vi "HAPS_PhaseSweep_Preamp(Hz).vi"() -> ()   [LabVIEW 2023, in "HAPS.lvlib"]
uses:
  HAPS.lvlib
  MCU_Function.ctl
  set_ele.ctl
  HAPS_SerialPort.ctl
  HAPS_MCU_ELE_Func.ctl
  R_S/R_S.lvlib
panel:
  in  "IC_On/OFF":bool[][](array[boolean])=[[TRUE, TRUE, TRUE, TRUE, TRUE, TRUE, FALSE, FALSE, FALSE, FALSE, FALSE, FALSE, TRUE], [FALSE, FALSE, FALSE, FALSE, FALSE, FALSE, FALSE, FALSE, FALSE, FALSE, FALSE, FALSE, FALSE], [FALSE, FALSE, FALSE, FALSE, FALSE, FALSE, TRUE, TRUE, TRUE, TRUE, TRUE, FALSE, TRUE]]
  in  "comn_gain":i32=17
  in  "ele_gain":i32=35
  in  "File_note":string
  in  "Init?":bool=TRUE
  out "Duration":dbl
  out "In-Phase : Phase(degree)":dbl[](graph)
  out "In-Phase : Gain(dB)":dbl[](graph)
  out "channel":i32
  out "chain_id":i32
  out "group":i32
  out "array_id":i32
  in  "Tx/Rx":enum16{"Rx", "Tx"}(ring)=enum."Tx"
  in  "array_id (MCU index)":i32
  in  "MCU_UART_addr":refnum<visa-resource-name>="COM8"
  in  "Target(degree)":dbl format="%#_13g"
  in  "SweepPoints":i32=11
  in  "sParameter":i32=21
  in  "Stop_Freq(GHz)":i64=39000000250
  in  "Start_Freq(GHz)":i64=38999999750
  in  "VISA resource name":refnum<visa-resource-name>="TCPIP0::192.168.119.45::inst0::INSTR"
  in  "HAPS_Equipment":enum16{"Keysight", "R&S"}(ring)=enum."R&S"
  # "HAPS_24x24_Phase_Sweep_Preamp(Hz)"
  # "VNA"
  # "DUT"
  # "Tx:35\nRx:22"
  # "4718.54"
  # "TCPIP0::192.168.1.31::hislip0::INSTR"
  # "Group_0"
  # "Group_1"
  # "Group_2"
  # "0"
  # "5"
  # "6"
  # "11"
  # "Test Status"
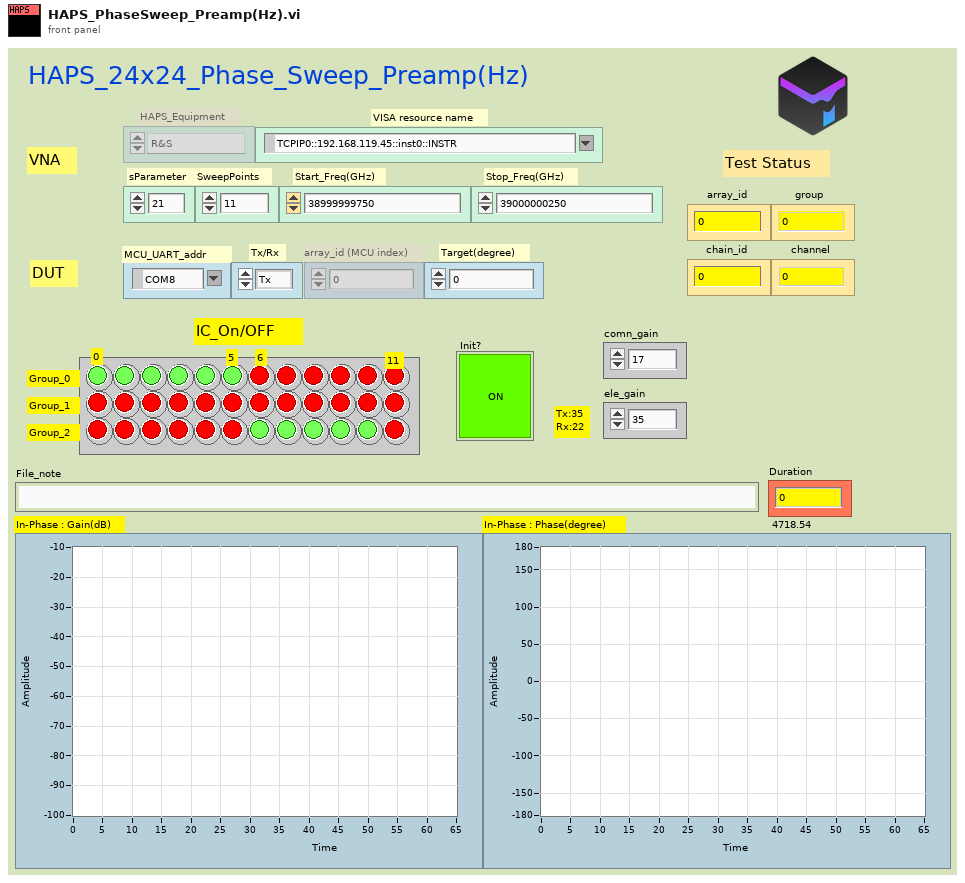
[diagram p1: front panel]
types:
  T1 = typedef "HAPS.lvlib/HAPS_SerialPort.ctl" = enum16{"Init", "Close", "CMD", "Flush"}
  T2 = typedef "HAPS.lvlib/HAPS_MCU_ELE_Func.ctl" = enum16{"array_init", "set_com_gain", "set_ch_gain_phase", "set_pd_range", "get_preamp_temp", "get_bfic_temp", "get_tx_pd", "ch_on", "ch_on_2", "ch_ctrl_all", "array_ctrl_src"}
  T3 = typedef "HAPS.lvlib/MCU_Function.ctl" = cluster{"Tx/Rx":enum16{"Rx", "Tx"}, "Enable?":enum16{"OFF", "On"}, "Source":enum16{"MCU", "ACU"}}
  T4 = typedef "HAPS.lvlib/set_ele.ctl" = cluster{"ch":i32, "chain_id":i32, "group":i32, "array_id":i32, "ele_phase":i32, "ele_gain":i32, "com_gain":i32, "pd_range":i32}
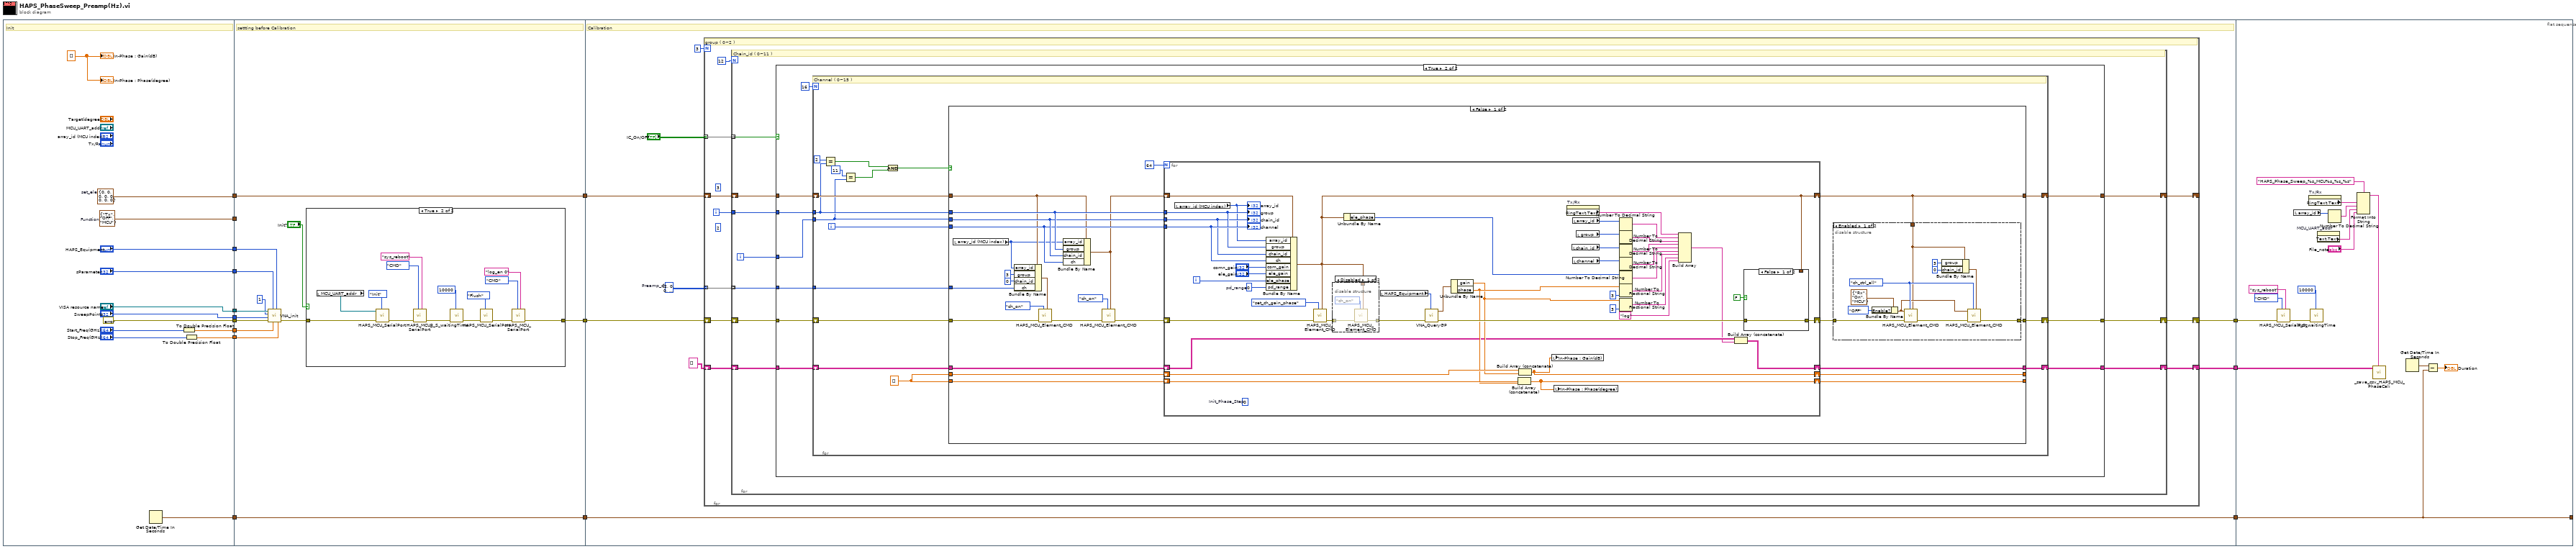
[diagram p0: block diagram]
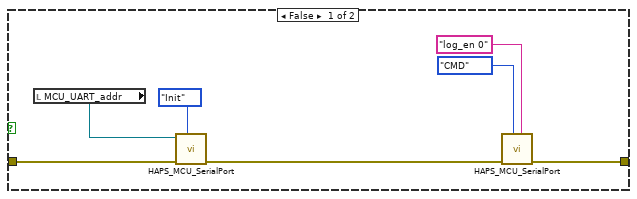
[diagram p2: hidden frame]
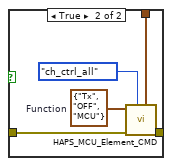
[diagram p6: hidden frame]
diagram:
  n1 = flat-sequence {
    tunnel: [w22] -> w16
    tunnel: [w29] -> w15
    tunnel: [errorcluster {"status"=FALSE, "code"=0, "source"=""} ("error in")] -> w13
    tunnel: ["sParameter"] -> w11
    tunnel: ["VISA resource name"] -> w10
    tunnel: [w18] -> w9
    tunnel: [w17] -> w8
    tunnel: ["SweepPoints"] -> w7
    tunnel: ["HAPS_Equipment"] -> w6
    tunnel: [w19] -> w4
    tunnel: w16 -> [w42]
    tunnel: w15 -> [_]
    tunnel: [w42] -> w14
    tunnel: w13 -> [w41]
    tunnel: [w33] -> w12
    tunnel: w11 -> [w40]
    tunnel: w10 -> [w39]
    tunnel: w9 -> [w38]
    tunnel: w8 -> [w37]
    tunnel: w7 -> [w36]
    tunnel: w6 -> [w32]
    tunnel: [w31] -> w5
    tunnel: w4 -> [w31]
    tunnel: w14 -> [w71]
    tunnel: w12 -> [w72]
    tunnel: w5 -> [w68]
    tunnel: [w68] -> w3
    tunnel: [w67] -> w2
    tunnel: [w65] -> w1
    tunnel: [w226] -> _
    tunnel: w3 -> [w226]
    tunnel: w2 -> [w228]
    tunnel: w1 -> [w221]
    frame #0 {
      w20 = dbl[] []
      w22 = T4 {"ch"=0, "chain_id"=0, "group"=0, "array_id"=0, "ele_phase"=0, "ele_gain"=0, "com_gain"=0, "pd_range"=0}  # set_ele
      w29 = T3 {"Tx/Rx"=enum."Tx", "Enable?"=enum."OFF", "Source"=enum."MCU"}  # Function
      # "Init"
      n2 = Get Date/Time In Seconds() -> (seconds since 1Jan1904=w19:timestamp)
      n3 = To Double Precision Float(number="Start_Freq(GHz)") -> (double precision float=w18:dbl)
      n4 = To Double Precision Float(number="Stop_Freq(GHz)") -> (double precision float=w17:dbl)
      "In-Phase : Gain(dB)" <- w20
      "In-Phase : Phase(degree)" <- w20
    }
    frame #1 {
      # "settting before Calibration"
      n5 = call "VNA_init.vi"("Stop_Freq(GHz)"=w37, "HAPS_MCU_CMD"=w32, "Start_Freq(GHz)"=w38, "sParameter"=w40, "error in"=w41, "SweepPoints"=w36, "Mark no."=1, "VISA resource name"=w39) -> ("error out"=w34:errorcluster)  [unwired: 3 in]
      n6 = case shown="True" "Init?" {
        tunnel: w34 -> [w47 w61]
        tunnel: [w44 w58] -> w33
        frame False {
          n7 = local read "MCU_UART_addr"() -> (w45:refnum<visa-resource-name>)
          n8 = call "HAPS_MCU_SerialPort.vi"("HAPS_SerialPort_Func"=HAPS_SerialPort."Init", "error in"=w47, "VISA resource name"=w45) -> ("error out"=w43:errorcluster)  [unwired: 6 in, 2 out]
          n9 = call "HAPS_MCU_SerialPort.vi"("Command"="log_en 0", "HAPS_SerialPort_Func"=enum16{"Init", "Close", "CMD"}."CMD" ("HAPS_SerialPort"), "error in"=w43) -> ("error out"=w44:errorcluster)  [unwired: 6 in, 2 out]
        }
        frame True {
          n10 = local read "MCU_UART_addr"() -> (w59:refnum<visa-resource-name>)
          n11 = call "HAPS_MCU_SerialPort.vi"("HAPS_SerialPort_Func"=HAPS_SerialPort."Init", "error in"=w61, "VISA resource name"=w59) -> ("error out"=w55:errorcluster)  [unwired: 6 in, 2 out]
          n12 = call "HAPS_MCU_SerialPort.vi"("Command"="sys_reboot", "HAPS_SerialPort_Func"=enum16{"Init", "Close", "CMD"}."CMD" ("HAPS_SerialPort"), "error in"=w55) -> ("error out"=w54:errorcluster)  [unwired: 6 in, 2 out]
          n13 = call "R_S_waitingTime.vi"("Waiting Time(ms)"=u32 10000, "error in"=w54) -> ("error out"=w52:errorcluster)  [unwired: 9 in]
          n14 = call "HAPS_MCU_SerialPort.vi"("HAPS_SerialPort_Func"=HAPS_SerialPort."Flush", "error in"=w52) -> ("error out"=w50:errorcluster)  [unwired: 7 in, 2 out]
          n15 = call "HAPS_MCU_SerialPort.vi"("Command"="log_en 0", "HAPS_SerialPort_Func"=enum16{"Init", "Close", "CMD"}."CMD" ("HAPS_SerialPort"), "error in"=w50) -> ("error out"=w58:errorcluster)  [unwired: 6 in, 2 out]
        }
      }
    }
    frame #2 {
      w66 = i32[][] [[2, 0, 0, 8, 8, 10, 11, 9, 9, 1, 1, 3], [3, 1, 1, 9, 9, 11, 13, 15, 15, 7, 7, 5], [5, 7, 7, 15, 15, 13, 14, 14, 6, 6, 4, 12]]  # Preamp_ch
      # "Calibration"
      n16 = for {
        N: 3 -> [_]
        shift-right: [w82] -> _
        shift-left: w71 -> [w78]
        shift-right: [w81] -> w67
        shift-left: string[][] [] -> [w77]
        shift-right: [w80] -> w65
        shift-left: w72 -> [w79]
        tunnel: w66 -> [w74] mode=indexing
        tunnel: "IC_On/OFF" -> [w73] mode=indexing
        i -> [w75]
        (unwired) 2
        (unwired) 3
        # "group ( 0~2 )"
        n17 = for {
          N: 12 -> [_]
          shift-right: [w92] -> w82
          shift-left: w78 -> [w89]
          shift-right: [w91] -> w81
          shift-left: w77 -> [w88]
          shift-right: [w85] -> w80
          shift-left: w79 -> [w90]
          tunnel: w75 -> [w87]
          tunnel: w74 -> [w84] mode=indexing
          tunnel: w73 -> [w83] mode=indexing
          i -> [w86]
          # "Chain_id ( 0~11 )"
          n18 = case shown="True" w83 {
            tunnel: [w93 w104] -> w92
            tunnel: [w95 w103] -> w91
            tunnel: w90 -> [w94 w102]
            tunnel: w89 -> [w93 w101]
            tunnel: w88 -> [w95 w100]
            tunnel: w87 -> [_ w99]
            tunnel: w86 -> [_ w98]
            tunnel: [w94 w97] -> w85
            tunnel: w84 -> [_ w96]
            frame False {
            }
            frame True {
              n19 = for {
                N: 16 -> [_]
                shift-right: [w118] -> w104
                shift-left: w101 -> [w121]
                shift-right: [w116] -> w103
                shift-left: w100 -> [w117]
                shift-right: [w119] -> w97
                shift-left: w102 -> [w120]
                tunnel: w99 -> [w115]
                tunnel: w98 -> [w107]
                tunnel: w96 -> [w106]
                i -> [w108]
                w109 = dbl[] []
                # "Channel ( 0~15 )"
                n20 = Equal?(x=2, y=w115) -> (x = y?=w112:bool)
                n21 = Equal?(x=11, y=w107) -> (x = y?=w111:bool)
                n22 = And(x=w112, y=w111) -> (x .and. y?=w110:bool)
                n23 = case shown="False" w110 {
                  tunnel: w121 -> [w128 w215]
                  tunnel: w108 -> [w137 _]
                  tunnel: w120 -> [w129 w214]
                  tunnel: w115 -> [w139 _]
                  tunnel: w107 -> [w138 _]
                  tunnel: w109 -> [w146 w217]
                  tunnel: w109 -> [w145 w218]
                  tunnel: [w144 w217] -> _
                  tunnel: [w143 w218] -> _
                  tunnel: [w133 w214] -> w119
                  tunnel: [w132 w215] -> w118
                  tunnel: w117 -> [w141 w216]
                  tunnel: [w140 w216] -> w116
                  tunnel: w106 -> [w122 _]
                  frame False {
                    n24 = local read "array_id (MCU index)"() -> (w126:i32)
                    n25 = Bundle By Name(cluster=w128, "array_id"=w126, "group"=3, "chain_id"=0, "ch"=w122) -> (w127:T4)
                    n26 = call "HAPS_MCU_Element_CMD.vi"("set_ele"=w127, "HAPS_MCU_ELE_Func."=HAPS_MCU_ELE_Func."ch_on", "error in"=w129) -> ("error out"=w130:errorcluster)  [unwired: 7 in, 1 out]
                    n27 = Bundle By Name(cluster=w128, "array_id"=w126, "group"=w139, "chain_id"=w138, "ch"=w137) -> (w123:T4)
                    n28 = call "HAPS_MCU_Element_CMD.vi"("set_ele"=w123, "HAPS_MCU_ELE_Func."=HAPS_MCU_ELE_Func."ch_on", "error in"=w130) -> ("error out"=w135:errorcluster)  [unwired: 7 in, 1 out]
                    n29 = for {
                      N: 64 -> [_]
                      tunnel: w137 -> [w201]
                      tunnel: w139 -> [w199]
                      tunnel: w138 -> [w198]
                      shift-right: [w174] -> w144
                      shift-left: w146 -> [w176]
                      shift-right: [w173] -> w143
                      shift-left: w145 -> [w175]
                      shift-right: [w170] -> w134
                      shift-left: w135 -> [w200]
                      shift-right: [w160] -> w132
                      shift-left: w123 -> [w202]
                      shift-right: [w164] -> w140
                      shift-left: w141 -> [w166]
                      i -> [w172]
                      w196 = 0  # pd_range
                      (unwired) 0  # Init_Phase_Step
                      n30 = local read "array_id (MCU index)"() -> (w194:i32)
                      "array_id" <- w194
                      n31 = Bundle By Name(cluster=w202, "array_id"=w194, "group"=w199, "chain_id"=w198, "ch"=w201, "com_gain"="comn_gain", "ele_gain"="ele_gain", "ele_phase"=w172, "pd_range"=w196) -> (w160:T4)
                      n32 = call "HAPS_MCU_Element_CMD.vi"("set_ele"=w160, "HAPS_MCU_ELE_Func."=HAPS_MCU_ELE_Func."set_ch_gain_phase", "error in"=w200) -> ("error out"=w162:errorcluster)  [unwired: 7 in, 1 out]
                      n33 = disable-structure shown="Disabled" {
                        disable-tunnel: w162 -> [w206 w207]
                        disable-tunnel: [w205 w207] -> w161
                        disable-tunnel: w160 -> [w203 _]
                        frame Disabled {
                          n34 = call "HAPS_MCU_Element_CMD.vi"("set_ele"=w203, "HAPS_MCU_ELE_Func."=HAPS_MCU_ELE_Func."ch_on", "error in"=w206) -> ("error out"=w205:errorcluster)  [unwired: 7 in, 1 out]
                        }
                        frame Enabled {
                        }
                      }
                      n35 = Unbundle By Name(w160) -> ("ele_phase"=w169:i32)
                      n36 = local read "HAPS_Equipment"() -> (w178:enum16{"Keysight", "R&S"})
                      n37 = call "VNA_QueryGP.vi"("HAPS_Equipment"=w178, "error in"=w161) -> ("error out"=w171:errorcluster, "queryMarker"=w177:cluster{"gain":dbl, "phase":dbl})  [unwired: 8 in]
                      n38 = Unbundle By Name(w177) -> ("gain"=w167:dbl, "phase"=w168:dbl)
                      n39 = Build Array (concatenate)(w175, w168) -> (w173:dbl[])
                      n40 = Build Array (concatenate)(w176, w167) -> (w174:dbl[])
                      n41 = local write "In-Phase : Gain(dB)"(w174) -> ()
                      n42 = local write "In-Phase : Phase(degree)"(w173) -> ()
                      n43 = property on="Tx/Rx" class="Enum (strict)"() -> ("RingText.Text"=w183:string)  [unwired: 2 in, 2 out]
                      n44 = local read "chain_id"() -> (w180:i32)
                      n45 = local read "array_id"() -> (w182:i32)
                      n46 = local read "channel"() -> (w179:i32)
                      n47 = local read "group"() -> (w181:i32)
                      n48 = Number To Decimal String(number=w182) -> (decimal integer string=w184:string)  [unwired: 1 in]
                      n49 = Number To Decimal String(number=w181) -> (decimal integer string=w185:string)  [unwired: 1 in]
                      n50 = Number To Decimal String(number=w180) -> (decimal integer string=w186:string)  [unwired: 1 in]
                      n51 = Number To Decimal String(number=w179) -> (decimal integer string=w187:string)  [unwired: 1 in]
                      n52 = Number To Decimal String(number=w169) -> (decimal integer string=w188:string)  [unwired: 1 in]
                      n53 = Number To Fractional String(number=w168, precision (6)=i16 3) -> (F-format string=w191:string)  [unwired: 2 in]
                      n54 = Number To Fractional String(number=w167, precision (6)=i16 3) -> (F-format string=w192:string)  [unwired: 2 in]
                      n55 = Build Array(w183, w184, w185, w186, w187, w188, w191, w192, "log") -> (w165:string[])
                      n56 = Build Array (concatenate)(w166, w165) -> (w164:string[][])
                      n57 = case shown="False" FALSE {
                        tunnel: w171 -> [w208 w211]
                        tunnel: [w208 w210] -> w170
                        tunnel: w160 -> [_ w209]
                        frame False {
                        }
                        frame True {
                          w213 = T3 {"Tx/Rx"=enum."Tx", "Enable?"=enum."OFF", "Source"=enum."MCU"}  # Function
                          n58 = call "HAPS_MCU_Element_CMD.vi"("set_ele"=w209, "HAPS_MCU_ELE_Func."=HAPS_MCU_ELE_Func."ch_ctrl_all", "error in"=w211, "Function"=w213) -> ("error out"=w210:errorcluster)  [unwired: 6 in, 1 out]
                        }
                      }
                      "group" <- w199
                      "chain_id" <- w198
                      "channel" <- w201
                    }
                    n59 = disable-structure shown="Enabled" {
                      disable-tunnel: w134 -> [w157 w158]
                      disable-tunnel: [w153 w158] -> w133
                      disable-tunnel: w132 -> [w147 _]
                      frame Enabled {
                        w152 = HAPS_MCU_ELE_Func."ch_ctrl_all" ("HAPS_MCU_ELE_Func.")
                        n60 = Bundle By Name(cluster=T3 {"Tx/Rx"=enum."Rx", "Enable?"=enum."On", "Source"=enum."MCU"} ("Function"), "Enable?"=enum16{"OFF", "On"}."OFF") -> (w151:T3)
                        n61 = call "HAPS_MCU_Element_CMD.vi"("set_ele"=w147, "HAPS_MCU_ELE_Func."=w152, "error in"=w157, "Function"=w151) -> ("error out"=w154:errorcluster)  [unwired: 6 in, 1 out]
                        n62 = Bundle By Name(cluster=w147, "group"=3, "chain_id"=0) -> (w148:T4)
                        n63 = call "HAPS_MCU_Element_CMD.vi"("set_ele"=w148, "HAPS_MCU_ELE_Func."=w152, "error in"=w154, "Function"=w151) -> ("error out"=w153:errorcluster)  [unwired: 6 in, 1 out]
                      }
                      frame Disabled {
                      }
                    }
                  }
                  frame True {
                  }
                }
              }
            }
          }
        }
      }
    }
    frame #3 {
      n64 = call "HAPS_MCU_SerialPort.vi"("Command"="sys_reboot", "HAPS_SerialPort_Func"=enum16{"Init", "Close", "CMD"}."CMD" ("HAPS_SerialPort"), "error in"=w221) -> ("error out"=w219:errorcluster)  [unwired: 6 in, 2 out]
      n65 = local read "array_id"() -> (w231:i32)
      n66 = property on="Tx/Rx" class="Enum (strict)"() -> ("RingText.Text"=w230:string)  [unwired: 2 in, 2 out]
      n67 = call "R_S_waitingTime.vi"("Waiting Time(ms)"=u32 10000, "error in"=w219) -> ()  [unwired: 9 in, 1 out]
      n68 = property on="MCU_UART_addr" class="VISAName"() -> ("Text.Text"=w234:string)  [unwired: 2 in, 2 out]
      n69 = Number To Decimal String(number=w231) -> (decimal integer string=w232:string)  [unwired: 1 in]
      n70 = Format Into String(format string="HAPS_Phase_Sweep_%s_MCU%s_%s_%s", w230, w232, w234, "File_note") -> (resulting string=w233:string)  [unwired: 2 in, 1 out]
      n71 = call "_save_csv_HAPS_MCU_PhaseCali.vi"("NoteName"=w233, "array in"=w228) -> ()  [unwired: 9 in, 1 out]
      n72 = Get Date/Time In Seconds() -> (seconds since 1Jan1904=w227:timestamp)
      n73 = Subtract(x=w227, y=w226) -> (x-y=→"Duration":dbl)
    }
  }
